vi "get_written_to_device.vi"(8 "error in (no error)":errorcluster, 11 "DAQmxWriteSignals in":refnum<class "SignalWriterMM140725DAQmx.lvclass">) -> (0 "error out":errorcluster, 2 "written to device?":bool, 3 "DAQmxWriteSignals out":refnum<class "SignalWriterMM140725DAQmx.lvclass">)   [LabVIEW 2010, in "SignalWriterMM140725DAQmx.lvclass"]
uses:
  SignalWriterMM140725DAQmx.lvclass
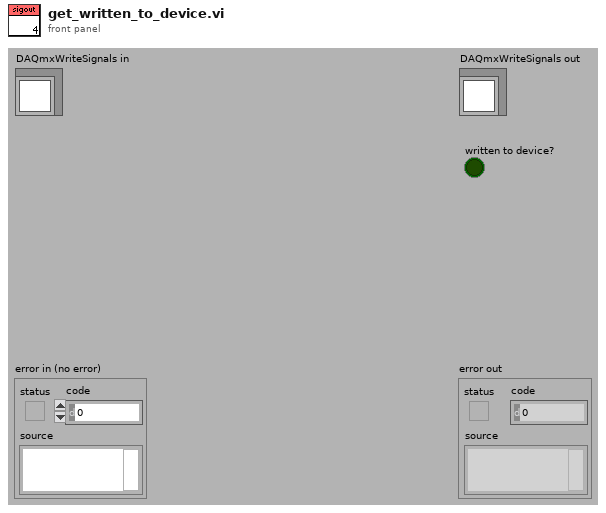
[diagram p1: front panel]
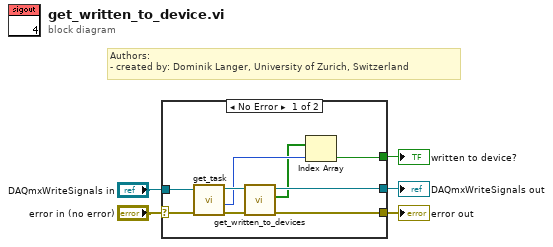
[diagram p0: block diagram]
diagram:
  # "Authors: \n- created by: Dominik Langer, University of Zurich, Switzerland"
  n1 = case shown="No Error" "error in (no error)" {
    selector: "error in (no error)" -> [w12 w16]
    tunnel: [w8 w16] -> w4
    tunnel: [w10 w15] -> w2
    tunnel: "DAQmxWriteSignals in" -> [w13 w15]
    tunnel: [w14 _] -> w1
    frame No Error {
      n2 = call-dynamic "get_task.vi"("error in (no error)"=w12, "DAQmxWriteSignals in"=w13) -> ("error out"=w9:errorcluster, "index"=w7:i32, "DAQmxWriteSignals out"=w11:refnum<class "SignalWriterMM140725DAQmx.lvclass">)  [unwired: 7 out]
      n3 = call-dynamic "get_written_to_devices.vi"("error in (no error)"=w9, "DAQmxWriteSignals in"=w11) -> ("error out"=w8:errorcluster, "written to devices?"=w6:bool[], "DAQmxWriteSignals out"=w10:refnum<class "SignalWriterMM140725DAQmx.lvclass">)  [unwired: 7 out]
      n4 = Index Array(array=w6, index=w7) -> (element=w14:bool)
    }
    frame Error {
    }
  }
  "error out" <- w4
  "DAQmxWriteSignals out" <- w2
  "written to device?" <- w1
